vi "Request.vi"(8 "error in":errorcluster, 10 "Request":T3, 11 "FINS Header i":T1={"resp req"=TRUE, "cmd resp"=FALSE, "SID"=0, "DNA"=0, "DA1"=10, "DA2"=0, "SA1"=0, "SA2"=251, "SNA"=0} {"SNA" max=127 format="%x"; "SA2" max=254 step=1 format="%x"; "SA1" format="%x"; "DA2" max=254 step=1 format="%x"; "DA1" format="%x"; "DNA" max=127 step=1 format="%x"}) -> (0 "error out":errorcluster={"status"=TRUE, "code"=0, "source"=""}, 1 "Paramters":string, 2 "FINS CMD":T2, 3 "FINS Header o":T1={"resp req"=TRUE, "cmd resp"=FALSE, "SID"=0, "DNA"=0, "DA1"=10, "DA2"=0, "SA1"=0, "SA2"=251, "SNA"=0} {"SNA" max=127 format="%x"; "SA2" max=254 step=1 format="%x"; "SA1" format="%x"; "DA2" max=254 step=1 format="%x"; "DA1" format="%x"; "DNA" max=127 step=1 format="%x"})   [LabVIEW 2019]
uses:
  Request.ctl
  FINS/FINS CMD.ctl
  FINS/FINS_header.ctl
  FINS/FINS CMD item.ctl
  FINS/FINS TCP.lvlib
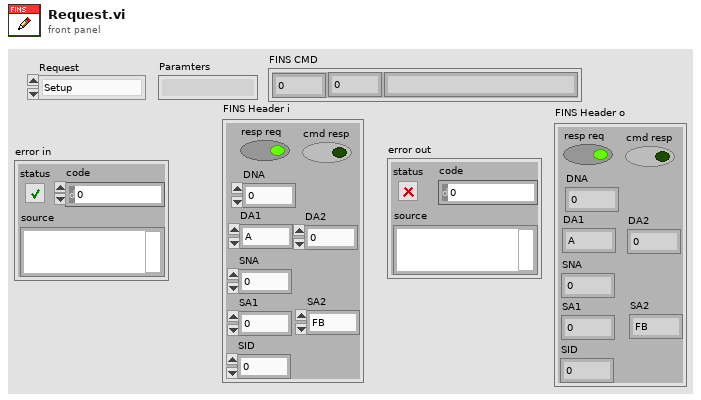
[diagram p1: front panel]
types:
  T1 = typedef "FINS TCP.lvlib/FINS_header.ctl" = cluster{"resp req":bool, "cmd resp":bool, "SID":u8, "DNA":u8, "DA1":u8, "DA2":u8, "SA1":u8, "SA2":u8, "SNA":u8}
  T2 = typedef "FINS TCP.lvlib/FINS CMD.ctl" = cluster{"MR":u8, "SR":u8, "name":string}
  T3 = typedef "Request.ctl" = enum16{"Setup", "Access Right: Acquire", "Access Right: Release", "STOP", "RUN", "Read_001", "Read_002", "Read_003", "Write_001"}
  T4 = typedef "FINS TCP.lvlib/FINS CMD item.ctl" = enum16{"FINS_UNKNOWN", "FINS_SETUP", "MEMORY AREA READ", "MEMORY AREA WRITE", "MEMORY AREA FILL", "MULTIPLE MEMORY AREA READ", "MEMORY AREA TRANSFER", "PARAMETER AREA READ", "PARAMETER AREA WRITE", "PARAMETER AREA CLEAR", "PROGRAM AREA PROTECT", "PROGRAM AREA PROTECT CLEAR", "PROGRAM AREA READ", "PROGRAM AREA WRITE", "PROGRAM AREA CLEAR", "RUN", "STOP", "CONTROLLER DATA READ", "CONNECTION DATA READ", "CONTROLLER STATUS READ", "CYCLE TIME READ", "CLOCK READ", "CLOCK WRITE", "MESSAGE READ", "MESSAGE CLEAR", "FAL/FALS READ", "ACCESS RIGHT ACQUIRE", "ACCESS RIGHT FORCED ACQUIRE", "ACCESS RIGHT RELEASE", "ERROR CLEAR", "ERROR LOG READ", "ERROR LOG CLEAR", "FILE NAME READ", "SINGLE FILE READ", "SINGLE FILE WRITE", "MEMORY CARD FORMAT", "FILE DELETE", "VOLUME LABEL CREATE/DELETE", "FILE COPY", "FILE NAME CHANGE", "FILE DATA CHECK", "MEMORY AREA FILE TRANSFER", "PARAMETER AREA FILE TRANSFER", "PROGRAM AREA FILE TRANSFER", "FORCED SET/RESET", "FORCED SET/RESET CANCEL"}
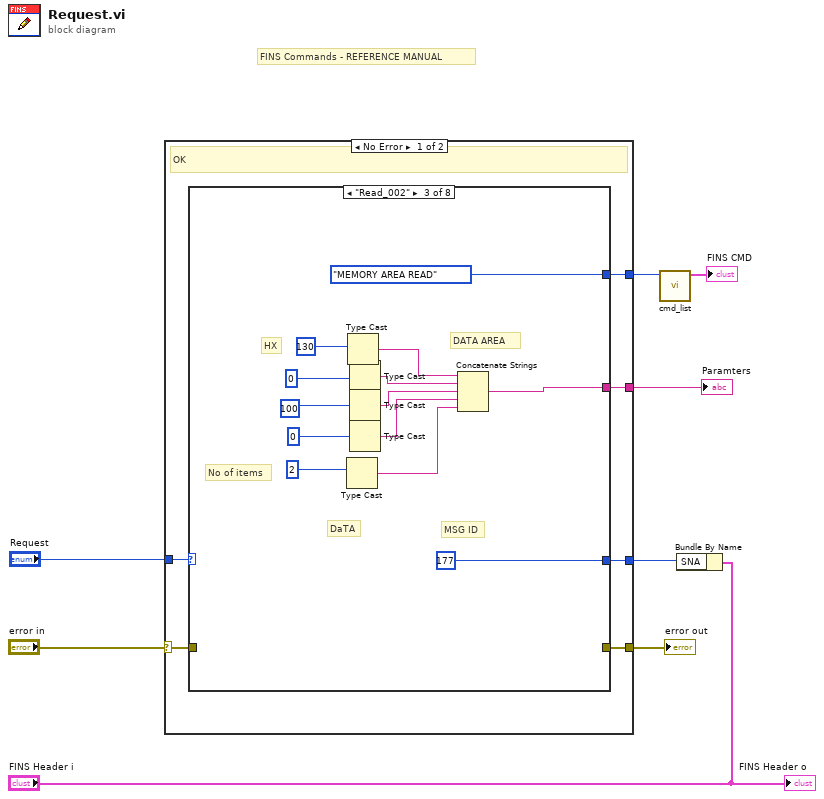
[diagram p0: block diagram]
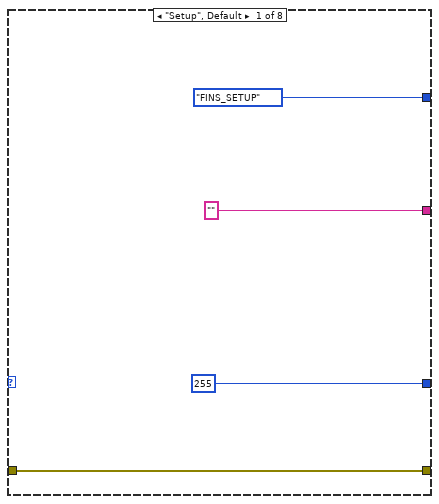
[diagram p2: hidden frame]
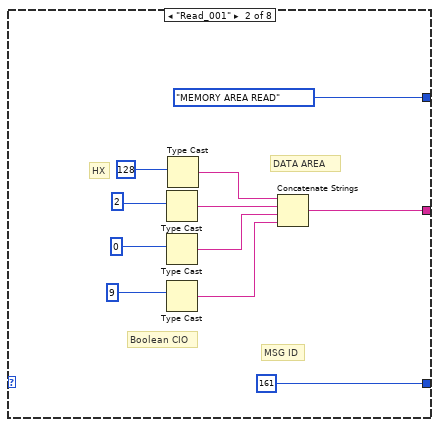
[diagram p3: hidden frame]
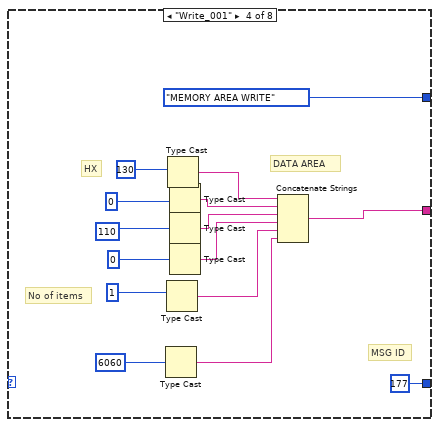
[diagram p4: hidden frame]
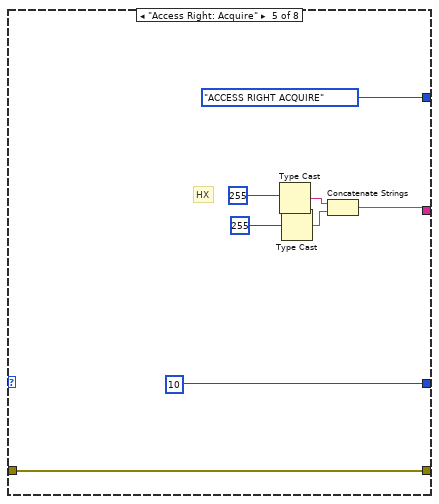
[diagram p5: hidden frame]
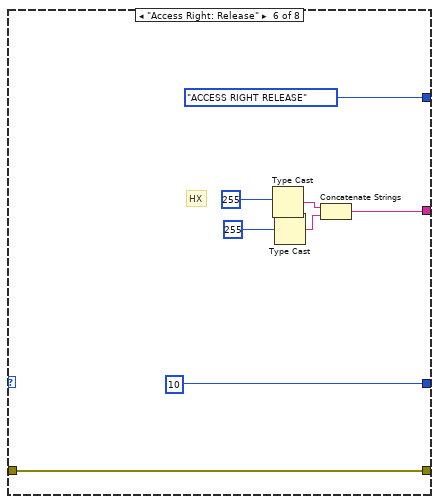
[diagram p6: hidden frame]
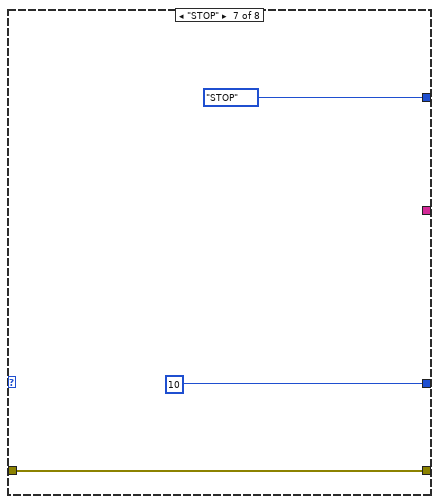
[diagram p7: hidden frame]
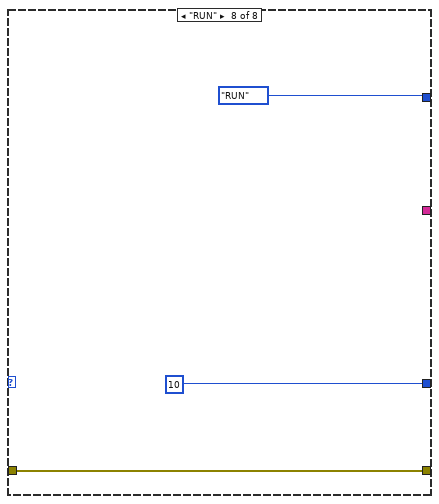
[diagram p8: hidden frame]
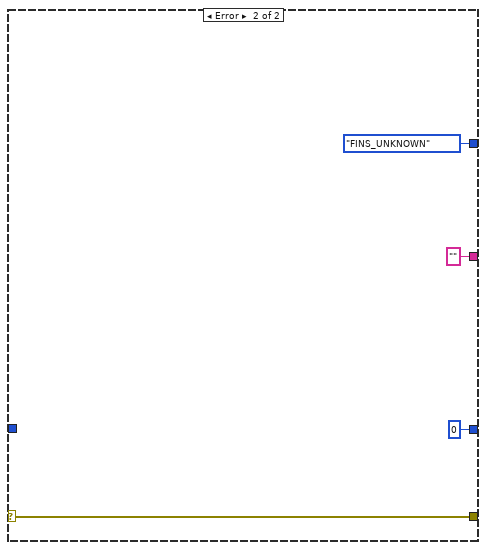
[diagram p9: hidden frame]
diagram:
  # "FINS Commands - REFERENCE MANUAL"
  n1 = case shown="No Error" "error in" {
    selector: "error in" -> [w10 w83]
    tunnel: [w14 ""] -> w8
    tunnel: [w13 u8 0 ("SNA")] -> w1
    tunnel: "Request" -> [w12 _]
    tunnel: [w11 w83] -> w6
    tunnel: [w9 FINS_CMD_item."FINS_UNKNOWN" ("CMD")] -> w3
    frame No Error {
      # "OK"
      n2 = case shown="\"Read_002\"" w12 {
        tunnel: ["" w21 w39 w54 w59 w67 _ _] -> w14
        tunnel: [u8 255 ("SNA") u8 161 ("SNA") u8 177 ("SNA") u8 177 ("SNA") u8 10 ("SNA") u8 10 ("SNA") u8 10 ("SNA") u8 10 ("SNA")] -> w13
        tunnel: w10 -> [w16 _ _ _ w65 w73 w76 w79]
        tunnel: [w16 _ _ _ w65 w73 w76 w79] -> w11
        tunnel: [FINS_CMD_item."FINS_SETUP" ("CMD") FINS_CMD_item."MEMORY AREA READ" ("CMD") FINS_CMD_item."MEMORY AREA READ" ("CMD") FINS_CMD_item."MEMORY AREA WRITE" ("CMD") FINS_CMD_item."ACCESS RIGHT ACQUIRE" ("CMD") FINS_CMD_item."ACCESS RIGHT RELEASE" ("CMD") FINS_CMD_item."STOP" ("CMD") FINS_CMD_item."RUN" ("CMD")] -> w9
        frame "Setup", Default {
        }
        frame "Read_001" {
          # "Boolean CIO"
          # "DATA AREA"
          # "MSG ID"
          # "HX"
          n3 = Type Cast(x=u16 2 ("length")) -> (*(type *) &x=w24:string)  [unwired: 1 in]
          n4 = Type Cast(x=u8 0 ("length")) -> (*(type *) &x=w23:string)  [unwired: 1 in]
          n5 = Type Cast(x=u16 9 ("length")) -> (*(type *) &x=w22:string)  [unwired: 1 in]
          n6 = Type Cast(x=u8 128 ("length")) -> (*(type *) &x=w25:string)  [unwired: 1 in]
          n7 = Concatenate Strings(w25, w24, w23, w22) -> (w21:string)
        }
        frame "Read_002" {
          # "No of items"
          # "DaTA"
          # "DATA AREA"
          # "MSG ID"
          # "HX"
          n8 = Type Cast(x=u16 2 ("length")) -> (*(type *) &x=w37:string)  [unwired: 1 in]
          n9 = Type Cast(x=u8 130 ("length")) -> (*(type *) &x=w40:string)  [unwired: 1 in]
          n10 = Type Cast(x=u8 0 ("length")) -> (*(type *) &x=w36:string)  [unwired: 1 in]
          n11 = Type Cast(x=u8 100 ("length")) -> (*(type *) &x=w35:string)  [unwired: 1 in]
          n12 = Type Cast(x=u8 0 ("length")) -> (*(type *) &x=w34:string)  [unwired: 1 in]
          n13 = Concatenate Strings(w40, w36, w35, w34, w37) -> (w39:string)
        }
        frame "Write_001" {
          # "No of items"
          # "DATA AREA"
          # "MSG ID"
          # "HX"
          n14 = Type Cast(x=u16 6060 ("length")) -> (*(type *) &x=w44:string)  [unwired: 1 in]
          n15 = Type Cast(x=u16 1 ("length")) -> (*(type *) &x=w52:string)  [unwired: 1 in]
          n16 = Type Cast(x=u8 130 ("length")) -> (*(type *) &x=w55:string)  [unwired: 1 in]
          n17 = Type Cast(x=u8 0 ("length")) -> (*(type *) &x=w51:string)  [unwired: 1 in]
          n18 = Type Cast(x=u8 110 ("length")) -> (*(type *) &x=w50:string)  [unwired: 1 in]
          n19 = Type Cast(x=u8 0 ("length")) -> (*(type *) &x=w49:string)  [unwired: 1 in]
          n20 = Concatenate Strings(w55, w51, w50, w49, w52, w44) -> (w54:string)
        }
        frame "Access Right: Acquire" {
          # "HX"
          n21 = Type Cast(x=u8 255 ("length")) -> (*(type *) &x=w63:string)  [unwired: 1 in]
          n22 = Type Cast(x=u8 255 ("length")) -> (*(type *) &x=w62:string)  [unwired: 1 in]
          n23 = Concatenate Strings(w63, w62) -> (w59:string)
        }
        frame "Access Right: Release" {
          # "HX"
          n24 = Type Cast(x=u8 255 ("length")) -> (*(type *) &x=w71:string)  [unwired: 1 in]
          n25 = Type Cast(x=u8 255 ("length")) -> (*(type *) &x=w70:string)  [unwired: 1 in]
          n26 = Concatenate Strings(w71, w70) -> (w67:string)
        }
        frame "STOP" {
        }
        frame "RUN" {
        }
      }
    }
    frame Error {
    }
  }
  "Paramters" <- w8
  "error out" <- w6
  n27 = call "cmd_list.vi"("CMD"=w3) -> ("cmd"=→"FINS CMD":T2)  [unwired: 9 in, 1 out]
  n28 = Bundle By Name(cluster="FINS Header i", "SNA"=w1) -> ()  [unwired: 1 out]
  "FINS Header o" <- "FINS Header i"
